vi "生成CODMn data (子VI).vi"() -> (3 "data":T1)   [LabVIEW 2016, in "斯坦道CODMn.lvlib"]
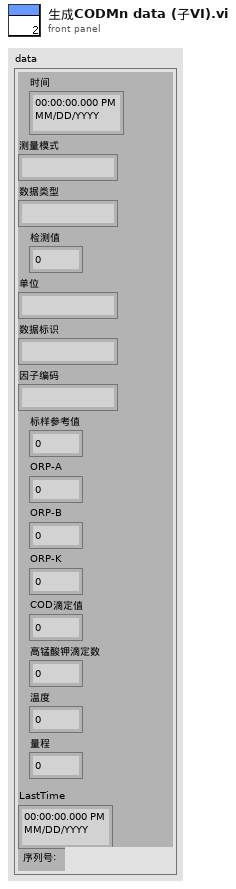
[diagram p1: front panel]
types:
  T1 = cluster{"时间":timestamp, "测量模式":string, "数据类型":string, "检测值":sgl, "单位":string, "数据标识":string, "因子编码":string, "标样参考值":sgl, "ORP-A":sgl, "ORP-B":sgl, "ORP-K":sgl, "COD滴定值":sgl, "高锰酸钾滴定数":sgl, "温度":sgl, "量程":sgl, "LastTime":timestamp, "序列号:":string}
  T2 = cluster{"运行模式":enum16{"维护模式", "常规模式", "应急模式", "质控模式"}, "质控频次":enum16{"关闭", "每天", "星期一", "星期二", "星期三", "星期四", "星期五", "星期六", "星期日"}, "空白核查时间":u16, "跨度核查时间":u16, "24H周期设置":bool[]}
  T3 = cluster{"测量量程":dbl, "测量精度":dbl, "测量间隔":dbl, "消解温度":dbl, "消解时长":dbl, "空白校准时间":timestamp, "曲线截距":dbl, "曲线斜率":dbl, "测量检出限":dbl, "测量信号值":dbl, "线性相关系数":dbl, "二次多项式系数":dbl, "标样校准时间":timestamp, "稀释倍数":dbl, "三项式系数":dbl, "空白标定系数":dbl, "量程系数":dbl, "F0/ORPA":dbl, "F1/ORPB":dbl, "F2/ORPK":dbl, "F3":dbl, "F4":dbl, "F5":dbl, "F6":dbl, "F7":dbl, "X0/滴定数":dbl, "量程":dbl}
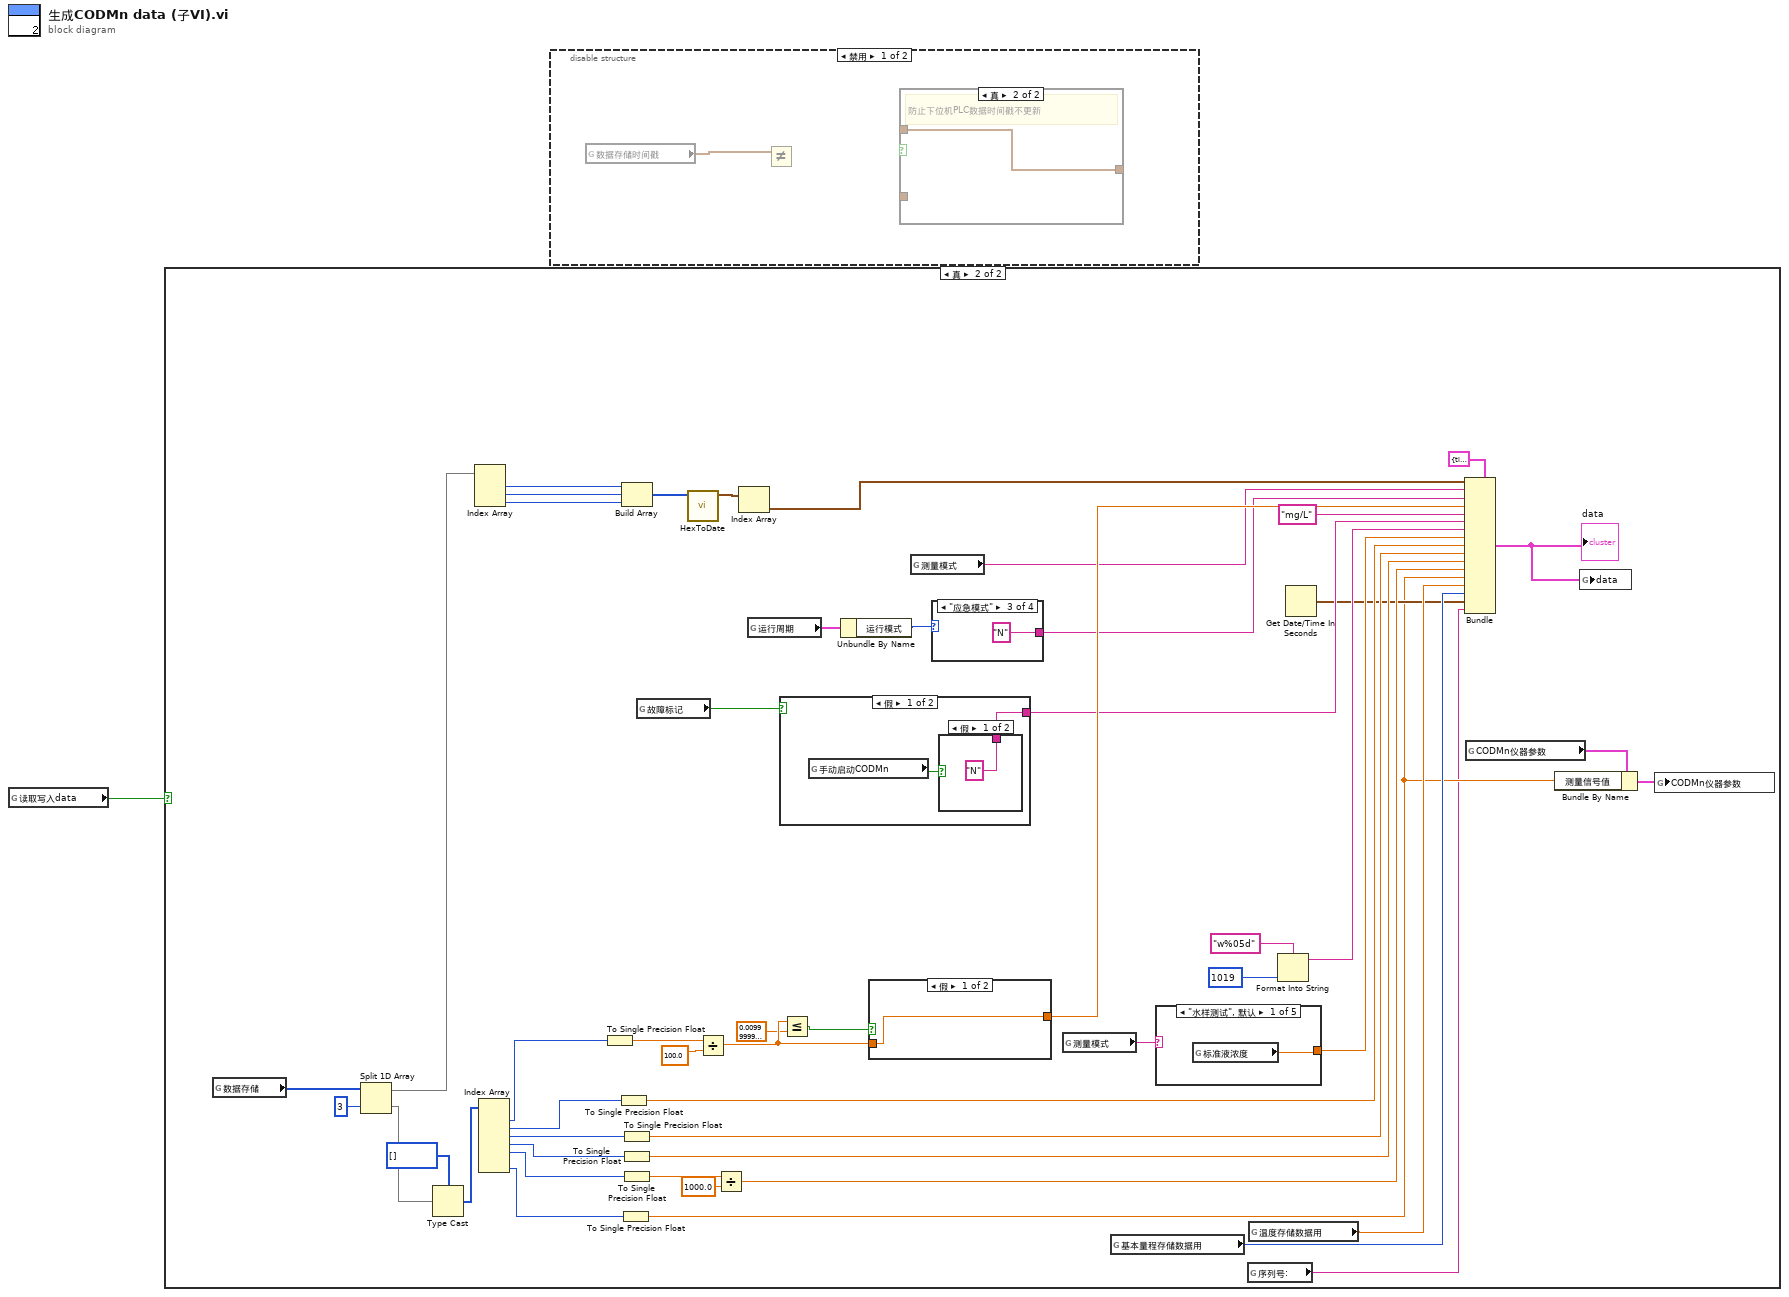
[diagram p0: block diagram]
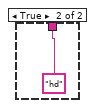
[diagram p5: hidden frame]
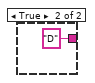
[diagram p6: hidden frame]
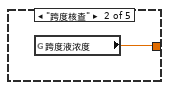
[diagram p7: hidden frame]
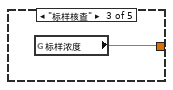
[diagram p8: hidden frame]
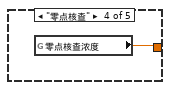
[diagram p9: hidden frame]
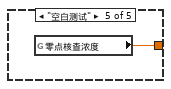
[diagram p10: hidden frame]
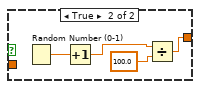
[diagram p11: hidden frame]
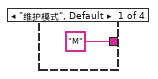
[diagram p12: hidden frame]
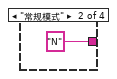
[diagram p13: hidden frame]
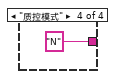
[diagram p14: hidden frame]
diagram:
  n1 = global read "COD内部交互全局.vi" "读取写入data"() -> (w1:bool)
  n2 = case shown="真" w1 {
    frame False {
    }
    frame True {
      n3 = global read "COD内部交互全局.vi" "数据存储"() -> (w12:u16[])
      n4 = Split 1D Array(array=w12, index=3 ("索引")) -> (first subarray=w17:u16[], second subarray=w11:u16[])
      n5 = Type Cast(type=i16[] [], x=w11) -> (*(type *) &x=w10:i16[])
      n6 = Index Array(array=w17) -> (element #1=w19:u16, element #2=w20:u16, element #3=w21:u16)  [unwired: 3 in]
      n7 = Index Array(array=w10) -> (element #1=w44:i16, element #2=w23:i16, element #3=w24:i16, element #4=w25:i16, element #5=w26:i16, element #7=w50:i16)  [unwired: 7 in, 1 out]
      n8 = To Single Precision Float(number=w44) -> (single precision float=w42:sgl)
      n9 = To Single Precision Float(number=w23) -> (single precision float=w35:sgl)
      n10 = To Single Precision Float(number=w50) -> (single precision float=w7:sgl)
      n11 = Build Array(w19, w20, w21) -> (w22:u16[])
      n12 = To Single Precision Float(number=w24) -> (single precision float=w34:sgl)
      n13 = To Single Precision Float(number=w25) -> (single precision float=w33:sgl)
      n14 = To Single Precision Float(number=w26) -> (single precision float=w29:sgl)
      n15 = global read "COD内部交互全局.vi" "故障标记"() -> (w52:bool)
      n16 = call "HexToDate.vi"("数组"=w22) -> ("DATE"=w18:timestamp[])  [unwired: 10 in]
      n17 = Divide(x=w42, y=sgl 100.0) -> (x/y=w43:sgl)
      n18 = Divide(x=w29, y=sgl 1000.0) -> (x/y=w32:sgl)
      n19 = Index Array(array=w18) -> (element=w6:timestamp)  [unwired: 1 in]
      n20 = global read "CODMn断电保存全局变量.vi" "运行周期"() -> (w2:T2)
      n21 = case shown="假" w52 {
        tunnel: [w54 "D" ("数据标识")] -> w37
        frame False {
          n22 = global read "CODMN外部API.vi" "手动启动CODMn"() -> (w53:bool)
          n23 = case shown="假" w53 {
            tunnel: ["N" ("数据标识") "hd" ("数据标识")] -> w54
            frame False {
            }
            frame True {
            }
          }
        }
        frame True {
        }
      }
      n24 = Less Or Equal?(x=w43, y=sgl 0.01) -> (x <= y?=w41:bool)
      n25 = Unbundle By Name(w2) -> ("运行模式"=w47:enum16{"维护模式", "常规模式", "应急模式", "质控模式"})
      n26 = case shown="假" w41 {
        tunnel: [w63 w64] -> w49
        tunnel: w43 -> [w63 _]
        frame False {
        }
        frame True {
          n27 = Random Number (0-1)() -> (number: 0 to 1=w67:dbl)
          n28 = Increment(x=w67) -> (x+1=w65:dbl)
          n29 = Divide(x=w65, y=sgl 100.0) -> (x/y=w64:dbl)
        }
      }
      n30 = global read "COD测量模式全局.vi" "测量模式"() -> (w48:string)
      n31 = case shown="\"应急模式\"" w47 {
        tunnel: ["M" ("单位") "N" ("单位") "N" ("单位") "N" ("单位")] -> w39
        frame "维护模式", Default {
        }
        frame "常规模式" {
        }
        frame "应急模式" {
        }
        frame "质控模式" {
        }
      }
      n32 = global read "COD测量模式全局.vi" "测量模式"() -> (w45:string)
      n33 = global read "COD内部交互全局.vi" "基本量程存储数据用"() -> (w15:enum16{"L", "H", "AUTO"})
      n34 = case shown="\"水样测试\", 默认" w45 {
        tunnel: [w58 w59 w60 w61 w62] -> w46
        frame "水样测试", Default {
          n35 = global read "COD浓度全局变量.vi" "标准液浓度"() -> (w58:dbl)
        }
        frame "跨度核查" {
          n36 = global read "CODMn断电保存全局变量.vi" "跨度液浓度"() -> (w59:dbl)
        }
        frame "标样核查" {
          n37 = global read "CODMn断电保存全局变量.vi" "标样浓度"() -> (w60:dbl)
        }
        frame "零点核查" {
          n38 = global read "CODMn断电保存全局变量.vi" "零点核查浓度"() -> (w61:dbl)
        }
        frame "空白测试" {
          n39 = global read "CODMn断电保存全局变量.vi" "零点核查浓度"() -> (w62:dbl)
        }
      }
      n40 = global read "COD内部交互全局.vi" "序列号:"() -> (w4:string)
      n41 = global read "COD内部交互全局.vi" "温度存储数据用"() -> (w51:dbl)
      n42 = Format Into String(format string="w%05d" ("格式字符串"), u32 1019 ("因子编码")) -> (resulting string=w36:string)  [unwired: 2 in, 1 out]
      n43 = Get Date/Time In Seconds() -> (seconds since 1Jan1904=w14:timestamp)
      n44 = Bundle(cluster=T1 {"时间"=timestamp(0 s since 1904-01-01), "测量模式"="", "数据类型"="", "检测值"=0.0, "单位"="", "数据标识"="", "因子编码"="", "标样参考值"=0.0, "ORP-A"=0.0, "ORP-B"=0.0, "ORP-K"=0.0, "COD滴定值"=0.0, "高锰酸钾滴定数"=0.0, "温度"=0.0, "量程"=0.0, "LastTime"=timestamp(0 s since 1904-01-01), "序列号:"=""} ("data"), "时间"=w6, "测量模式"=w48, "数据类型"=w39, "检测值"=w49, "单位"="mg/L", "数据标识"=w37, "因子编码"=w36, "标样参考值"=w46, "ORP-A"=w35, "ORP-B"=w34, "ORP-K"=w33, "COD滴定值"=w32, "高锰酸钾滴定数"=w7, "温度"=w51, "量程"=w15, "LastTime"=w14, "序列号:"=w4) -> (w3:T1)
      "data" <- w3
      n45 = global read "CODMn断电保存全局变量.vi" "CODMn仪器参数"() -> (w9:T3)
      n46 = Bundle By Name(cluster=w9, "测量信号值"=w7) -> (w8:T3)
      n47 = global write "COD内部交互全局.vi" "data"(w3) -> ()
      n48 = global write "CODMn断电保存全局变量.vi" "CODMn仪器参数"(w8) -> ()
    }
  }
  n49 = disable-structure shown="禁用" {
    frame Disabled {
      n50 = global read "COD内部交互全局.vi" "数据存储时间戳"() -> (w72:timestamp)
      n51 = Not Equal?(x=w72) -> (x != y?=w73:bool)  [unwired: 1 in]
      n52 = case "条件结构" shown="真" {
        selector: _ -> [_ _]
        tunnel: _ -> [w74 _]
        tunnel: _ -> [_ w75]
        tunnel: [w74 w75] -> _
        frame False {
        }
        frame True {
          # "防止下位机PLC数据时间戳不更新"
        }
      }
    }
    frame Enabled {
    }
  }
